vi "Grid FormatString.vi"(9 "文字列":string, 11 "Control入力":refnum<vi>) -> (1 "フォーマット後文字列":string)   [LabVIEW 2014]
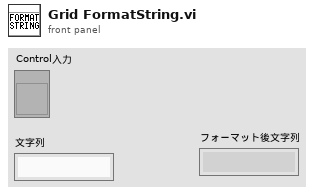
[diagram p1: front panel]
types:
  T1 = typedef "Clust ClassID.ctl" = enum16{"０", "１", "２", "３", "４", "５", "６", "色", "ブール", "９", "１０", "パス", "１２", "１３", "配列", "１５", "１６", "１７", "数値", "１９", "２０", "２１", "２２", "２３", "２４", "２５", "２６", "文字列", "２８", "２９", "３０", "３１", "３２", "３３", "リング", "Enum", "３６"}
  T2 = typedef "LVMinMaxIncTypeDef.ctl" = cluster{"Minimum":dbl, "Maximum":dbl, "Increment":dbl}
  T3 = typedef "LVStringsAndValuesArrayTypeDef.ctl" = cluster{"String":string, "Value":ext}[]
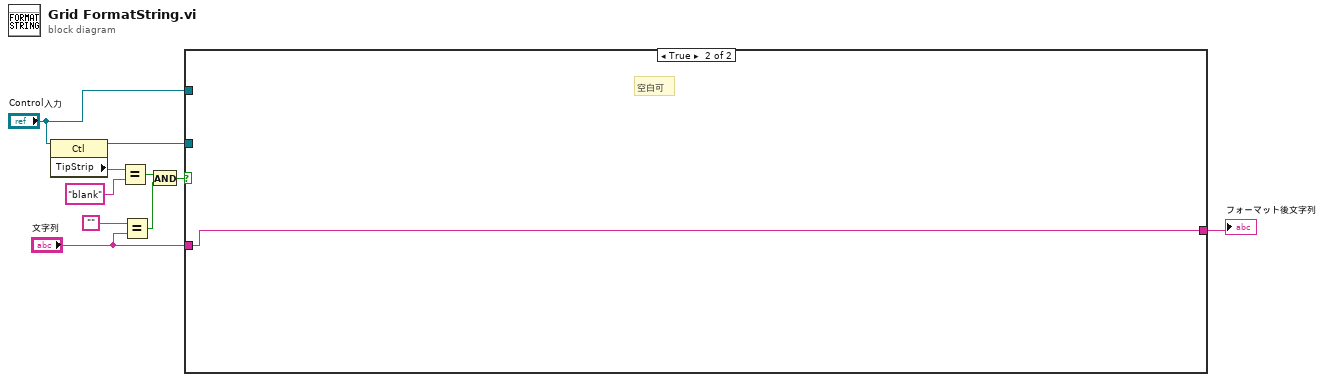
[diagram p0: block diagram]
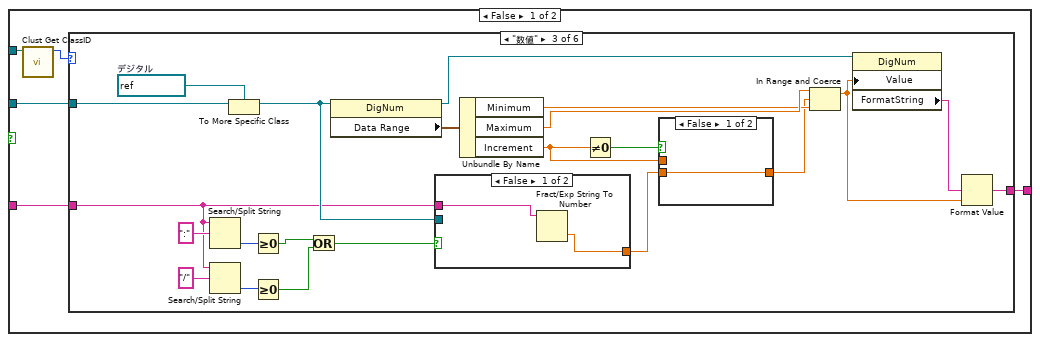
[diagram p2: hidden frame]
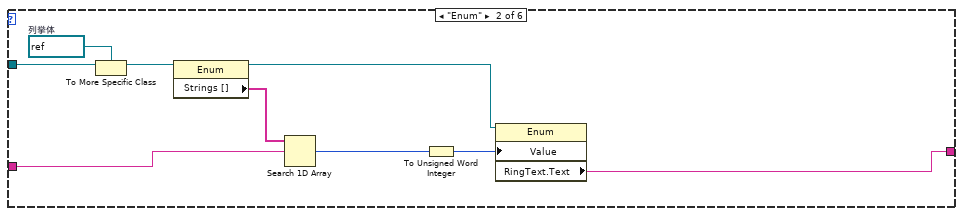
[diagram p4: hidden frame]
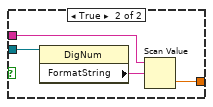
[diagram p5: hidden frame]
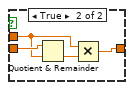
[diagram p6: hidden frame]
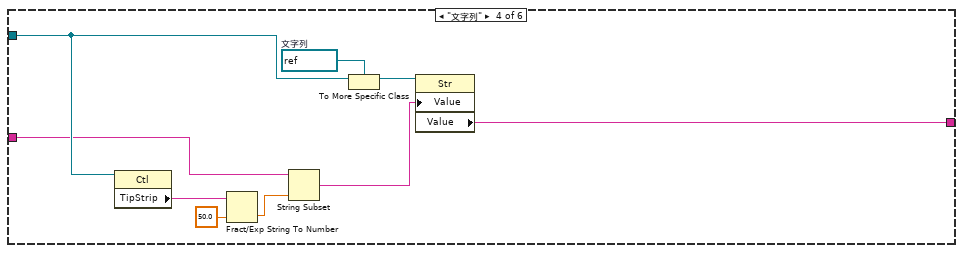
[diagram p7: hidden frame]
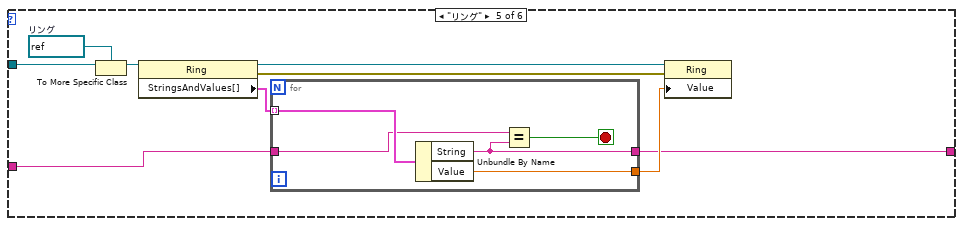
[diagram p8: hidden frame]
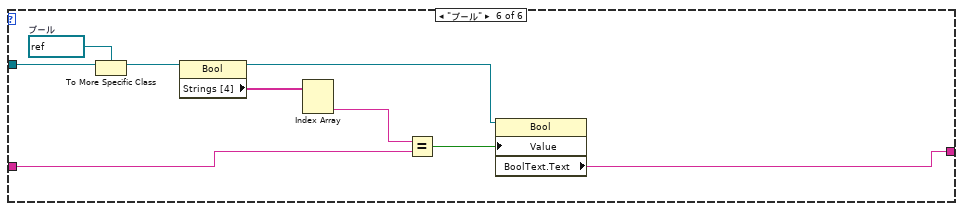
[diagram p9: hidden frame]
diagram:
  n1 = property class="Ctl"(reference="Control入力") -> (reference out=w9:refnum<vi>, "TipStrip"=w7:string)  [unwired: 1 in, 1 out]
  n2 = Equal?(x=w7, y="blank") -> (x = y?=w3:bool)
  n3 = Equal?(x="", y="文字列") -> (x = y?=w2:bool)
  n4 = And(x=w3, y=w2) -> (x .and. y?=w1:bool)
  n5 = case shown="TRUE" w1 {
    tunnel: [w15 w91] -> w10
    tunnel: w9 -> [w13 _]
    tunnel: "Control入力" -> [w12 _]
    tunnel: "文字列" -> [w11 w91]
    frame False {
      n6 = call "Clust Get ClassID.vi"("Ctl Refnum"=w12) -> ("ClassID"=w14:T1)  [unwired: 10 in]
      n7 = case shown="\"数値\"" w14 {
        tunnel: [w16 w17 w47 w67 w68 w82] -> w15
        tunnel: w13 -> [_ w24 w37 w64 w75 w89]
        tunnel: w11 -> [w16 w21 w30 w59 w71 w84]
        frame Default {
        }
        frame "Enum" {
          w25 = refnum<vi> refnum  # 列挙体
          n8 = To More Specific Class(target class=w25, reference=w24) -> (specific class reference=w23:refnum<vi>)  [unwired: 1 in, 1 out]
          n9 = property class="Enum"(reference=w23) -> (reference out=w19:refnum<vi>, "Strings []"=w22:string[])  [unwired: 1 in, 1 out]
          n10 = Search 1D Array(1D array=w22, element=w21) -> (index of element=w20:i32)  [unwired: 1 in]
          n11 = To Unsigned Word Integer(number=w20) -> (unsigned 16bit integer=w18:u16)
          n12 = property class="Enum"(reference=w19, "Value"=w18) -> ("RingText.Text"=w17:string)  [unwired: 1 in, 2 out]
        }
        frame "数値" {
          w38 = refnum<vi> refnum  # デジタル
          n13 = Search/Split String(string=w30, search string/char (-)=":" ("検索文字列／文字 （-）")) -> (offset of match=w32:i32)  [unwired: 1 in, 2 out]
          n14 = Search/Split String(string=w30, search string/char (-)="/" ("検索文字列／文字 （-）")) -> (offset of match=w29:i32)  [unwired: 1 in, 2 out]
          n15 = To More Specific Class(target class=w38, reference=w37) -> (specific class reference=w34:refnum<vi>)  [unwired: 1 in, 1 out]
          n16 = Greater Or Equal To 0?(x=w32) -> (x >= 0?=w27:bool)
          n17 = Greater Or Equal To 0?(x=w29) -> (x >= 0?=w26:bool)
          n18 = Or(x=w27, y=w26) -> (x .or. y?=w28:bool)
          n19 = property class="DigNum"(reference=w34) -> (reference out=w41:refnum<vi>, "Data Range"=w46:T2)  [unwired: 1 in, 1 out]
          n20 = case shown="FALSE" w28 {
            tunnel: [w48 w53] -> w45
            tunnel: w34 -> [_ w52]
            tunnel: w30 -> [w49 w50]
            frame False {
              n21 = Fract/Exp String To Number(string=w49) -> (number=w48:dbl)  [unwired: 3 in, 1 out]
            }
            frame True {
              n22 = property class="DigNum"(reference=w52) -> ("FormatString"=w51:string)  [unwired: 1 in, 2 out]
              n23 = Scan Value(string=w50, format string=w51) -> (value=w53:dbl)  [unwired: 1 in, 1 out]
            }
          }
          n24 = Unbundle By Name(w46) -> ("Minimum"=w43:dbl, "Maximum"=w44:dbl, "Increment"=w36:dbl)
          n25 = Not Equal To 0?(x=w36) -> (x != 0?=w35:bool)
          n26 = case shown="FALSE" w35 {
            tunnel: w45 -> [w54 w58]
            tunnel: [w54 w56] -> w42
            tunnel: w36 -> [_ w55]
            frame False {
            }
            frame True {
              n27 = Quotient & Remainder(x=w58, y=w55) -> (floor(x/y)=w57:dbl)  [unwired: 1 out]
              n28 = Multiply(x=w55, y=w57) -> (x*y=w56:dbl)
            }
          }
          n29 = In Range and Coerce(upper limit=w44, x=w42, lower limit=w43) -> (coerced(x)=w40:dbl)  [unwired: 1 out]
          n30 = property class="DigNum"(reference=w41, "Value"=w40) -> ("FormatString"=w39:string)  [unwired: 1 in, 2 out]
          n31 = Format Value(format string=w39, value (0)=w40) -> (output string=w47:string)  [unwired: 1 in]
        }
        frame "文字列" {
          w66 = refnum<vi> refnum  # 文字列
          n32 = property class="Ctl"(reference=w64) -> ("TipStrip"=w62:string)  [unwired: 1 in, 2 out]
          n33 = Fract/Exp String To Number(string=w62, default (0 dbl)=50.0 ("デフォルト （0 DBL）")) -> (number=w61:dbl)  [unwired: 2 in, 1 out]
          n34 = String Subset(string=w59, length (rest)=w61) -> (substring=w60:string)  [unwired: 1 in]
          n35 = To More Specific Class(target class=w66, reference=w64) -> (specific class reference=w65:refnum<vi>)  [unwired: 1 in, 1 out]
          n36 = property class="Str"(reference=w65, "Value"=w60) -> ("Value"=w67:string)  [unwired: 1 in, 2 out]
        }
        frame "リング" {
          w74 = refnum<vi> refnum  # リング
          n37 = To More Specific Class(target class=w74, reference=w75) -> (specific class reference=w73:refnum<vi>)  [unwired: 1 in, 1 out]
          n38 = property class="Ring"(reference=w73) -> (reference out=w76:refnum<vi>, error out=w69:errorcluster, "StringsAndValues[]"=w72:T3)  [unwired: 1 in]
          n39 = for {
            tunnel: w72 -> [w81] mode=indexing
            tunnel: w71 -> [w80]
            tunnel: [w78] -> w68
            tunnel: [w77] -> w70
            stop <- w79 stop-if-true
            n40 = Unbundle By Name(w81) -> ("String"=w78:string, "Value"=w77:ext)
            n41 = Equal?(x=w80, y=w78) -> (x = y?=w79:bool)
          }
          n42 = property class="Ring"(reference=w76, error in=w69, "Value"=w70) -> ()  [unwired: 2 out]
        }
        frame "ブール" {
          w90 = refnum<vi> refnum  # ブール
          n43 = To More Specific Class(target class=w90, reference=w89) -> (specific class reference=w88:refnum<vi>)  [unwired: 1 in, 1 out]
          n44 = property class="Bool"(reference=w88) -> (reference out=w87:refnum<vi>, "Strings [4]"=w86:string[])  [unwired: 1 in, 1 out]
          n45 = Index Array(array=w86) -> (element #2=w85:string)  [unwired: 2 in, 1 out]
          n46 = Equal?(x=w85, y=w84) -> (x = y?=w83:bool)
          n47 = property class="Bool"(reference=w87, "Value"=w83) -> ("BoolText.Text"=w82:string)  [unwired: 1 in, 2 out]
        }
      }
    }
    frame True {
      # "空白可"
    }
  }
  "フォーマット後文字列" <- w10
